vi "SubVI_TurnLeft_Auto.vi"(10 "Speed":dbl=1000.0) -> ()   [LabVIEW 2017]
uses:
  <vilib>/Rock Robotics/WPI/ThirdParty/Sensors/navX/_TypeDefs/FRIC_navX_DeviceNumbersTypeDef.ctl
  <vilib>/Rock Robotics/WPI/ThirdParty/Phoenix-LabVIEW/Motor Controller/Controls/CTRE_Phoenix_MotorControl_ControlMode.ctl
panel:
  out "Yaw":dbl
  in  "F 2":dbl=0.1
  in  "D 2":dbl=0.1
  in  "I 2":dbl
  in  "P 2":dbl=0.025
  in  "F":dbl=0.1
  in  "D":dbl=0.1
  in  "I":dbl
  in  "P":dbl=0.025
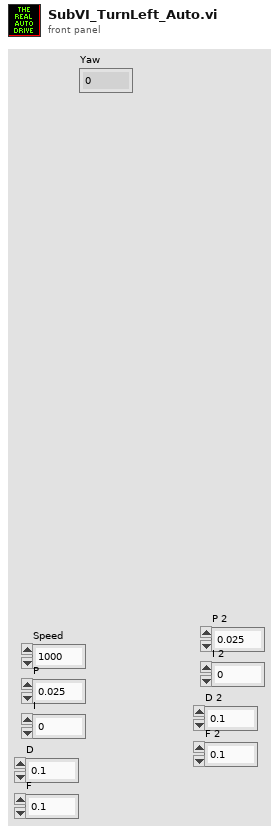
[diagram p1: front panel]
types:
  T1 = typedef "FRIC_navX_DeviceNumbersTypeDef.ctl" = enum16{"Dev0", "Dev1", "Dev2", "Dev3"}
  T2 = typedef "WPI_MotorControlDeviceRef.ctl" = cluster{"DeviceStatus":errorcluster, "Type":T3, "PWM":cluster{"PWM Channel":T4, "DeadBand":T5}, "CAN":cluster{"Device Number":u8, "SetOutput VI Ref":variant, "GetOutput VI Ref":variant, "Enable VI Ref":variant, "Disable VI Ref":variant, "Data":variant}, "Invert":bool, "DIO PWM":cluster{"PWM \"Enable\" Channel":T4, "DIOChannel":T6, "PWM Rate":dbl}}
  T3 = typedef "WPI_MotorControlType.ctl" = enum16{"PWM", "CAN", "DIO PWM"}
  T4 = typedef "FPGA_DIOPWMChannel.ctl" = enum8{"PWM 0", "PWM 1", "PWM 2", "PWM 3", "PWM 4", "PWM 5", "PWM 6", "PWM 7", "PWM 8", "PWM 9", "PWM MXP 0", "PWM MXP 1", "PWM MXP 2", "PWM MXP 3", "PWM MXP 4", "PWM MXP 5", "PWM MXP 6", "PWM MXP 7", "PWM MXP 8", "PWM MXP 9", "Invalid"}
  T5 = typedef "WPI_PWMDeadband.ctl" = cluster{"Name":string, "maxPositivePwm":i32, "minPositivePwm":i32, "centerPwm":i32, "maxNegativePwm":i32, "minNegativePwm":i32, "angularRange":u16}
  T6 = typedef "FPGA_DIOChannel.ctl" = enum8{"DIO 0", "DIO 1", "DIO 2", "DIO 3", "DIO 4", "DIO 5", "DIO 6", "DIO 7", "DIO 8", "DIO 9", "DIO MXP 0", "DIO MXP 1", "DIO MXP 2", "DIO MXP 3", "DIO MXP 4", "DIO MXP 5", "DIO MXP 6", "DIO MXP 7", "DIO MXP 8", "DIO MXP 9", "DIO MXP 10", "DIO MXP 11", "DIO MXP 12", "DIO MXP 13", "DIO MXP 14", "DIO MXP 15", "SPI Port CS1", "SPI Port CS2", "SPI Port CS3", "SPI Port MISO", "SPI Port MOSI", "Invalid"}
  T7 = cluster{"Yaw":dbl, "Roll":dbl, "Pitch":dbl, "Heading":dbl, "Fused Heading":dbl}
  T8 = typedef "CTRE_Phoenix_MotorControl_ControlMode.ctl" = u16
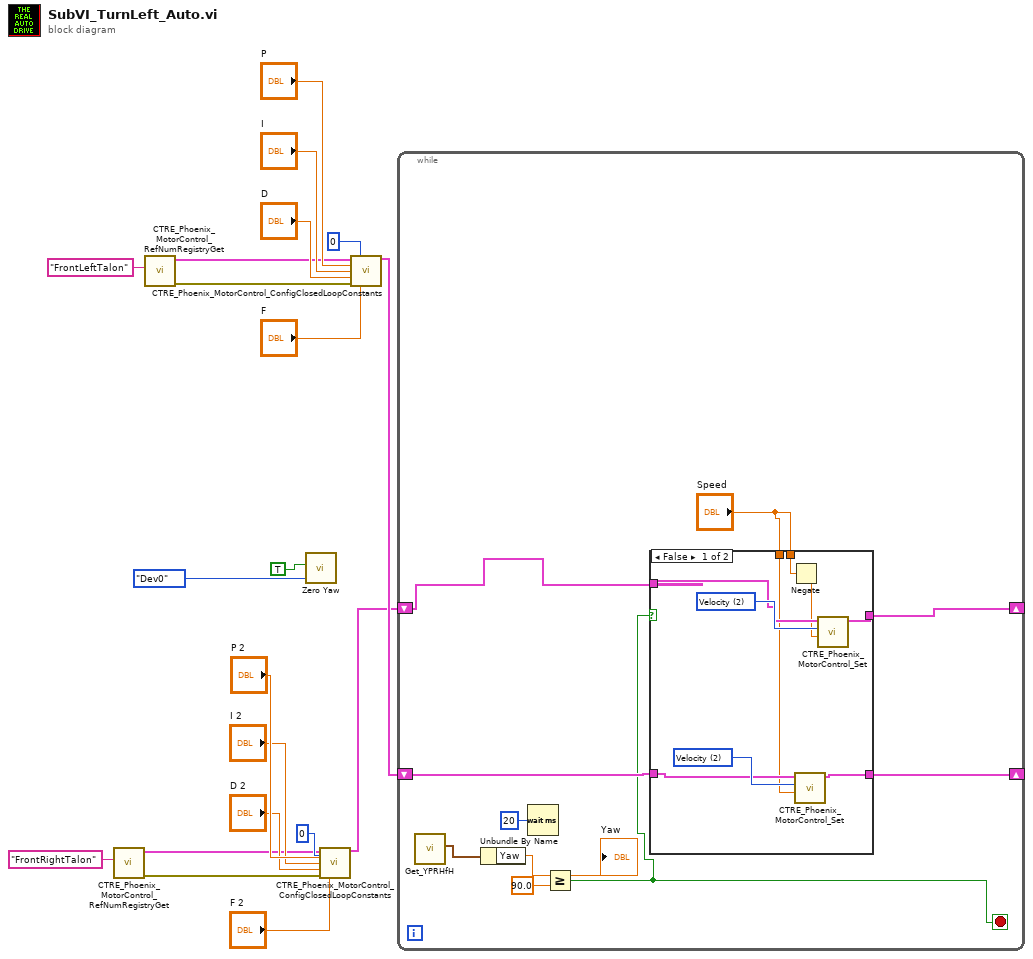
[diagram p0: block diagram]
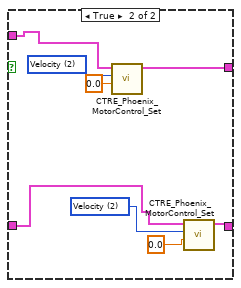
[diagram p2: hidden frame]
diagram:
  n1 = call <vilib>:"CTRE_Phoenix_MotorControl_RefNumRegistryGet.vi"("refnum name"="FrontRightTalon") -> ("error out"=w3:errorcluster, "PhoenixMotorControlDevRef"=w4:T2)  [unwired: 9 in]
  n2 = call <vilib>:"CTRE_Phoenix_MotorControl_RefNumRegistryGet.vi"("refnum name"="FrontLeftTalon") -> ("error out"=w5:errorcluster, "PhoenixMotorControlDevRef"=w6:T2)  [unwired: 9 in]
  n3 = call <vilib>:"Zero Yaw.vi"("Device Number"=FRIC_navX_DeviceNumbersTypeDef."Dev0", "Zero"=TRUE) -> ()  [unwired: 10 in]
  n4 = call <vilib>:"CTRE_Phoenix_MotorControl_ConfigClosedLoopConstants.vi"("PhoenixMotorControlDevRef"=w4, "slotIdx"=0, "P"="P 2", "I"="I 2", "D"="D 2", "error in (no error)"=w3, "F"="F 2") -> ("PhoenixMotorControlDevRef"=w7:T2)  [unwired: 7 in, 1 out]
  n5 = call <vilib>:"CTRE_Phoenix_MotorControl_ConfigClosedLoopConstants.vi"("PhoenixMotorControlDevRef"=w6, "slotIdx"=0, "P"="P", "I"="I", "D"="D", "error in (no error)"=w5, "F"="F") -> ("PhoenixMotorControlDevRef"=w16:T2)  [unwired: 7 in, 1 out]
  n6 = while {
    shift-right: [w23] -> _
    shift-left: w16 -> [w24]
    shift-right: [w30] -> _
    shift-left: w7 -> [w28]
    stop <- w22 stop-if-true
    n7 = call <vilib>:"Get_YPRHfH.vi"() -> ("YRPHfH"=w27:T7)  [unwired: 11 in]
    n8 = Unbundle By Name(w27) -> ("Yaw"=w26:dbl)
    "Yaw" <- w26
    n9 = Wait (ms)(milliseconds to wait=u32 20) -> ()  [unwired: 1 out]
    n10 = Greater Or Equal?(x=w26, y=90.0) -> (x >= y?=w22:bool)
    n11 = case shown="False" w22 {
      tunnel: [w38 w45] -> w30
      tunnel: w28 -> [w37 w44]
      tunnel: w24 -> [w35 w42]
      tunnel: [w34 w40] -> w23
      tunnel: "Speed" -> [w33 _]
      tunnel: "Speed" -> [w31 _]
      frame False {
        w36 = T8 2 items=["PercentOutput"=0, "Position"=1, "Velocity"=2, "Current"=3, "Follower"=5, "MotionProfile"=6, "MotionMagic"=7, "MotionMagicArc"=8, "MotionProfileArc"=10, "Disabled"=15] ("Control Mode")
        w39 = T8 2 items=["PercentOutput"=0, "Position"=1, "Velocity"=2, "Current"=3, "Follower"=5, "MotionProfile"=6, "MotionMagic"=7, "MotionMagicArc"=8, "MotionProfileArc"=10, "Disabled"=15] ("Control Mode")
        n12 = Negate(x=w33) -> (-x=w32:dbl)
        n13 = call <vilib>:"CTRE_Phoenix_MotorControl_Set.vi"("Output"=w31, "Control Mode"=w36, "PhoenixMotorControlDevRef"=w35) -> ("PhoenixMotorControlDevRef"=w34:T2)  [unwired: 7 in, 1 out]
        n14 = call <vilib>:"CTRE_Phoenix_MotorControl_Set.vi"("Output"=w32, "Control Mode"=w39, "PhoenixMotorControlDevRef"=w37) -> ("PhoenixMotorControlDevRef"=w38:T2)  [unwired: 7 in, 1 out]
      }
      frame True {
        w43 = T8 2 items=["PercentOutput"=0, "Position"=1, "Velocity"=2, "Current"=3, "Follower"=5, "MotionProfile"=6, "MotionMagic"=7, "MotionMagicArc"=8, "MotionProfileArc"=10, "Disabled"=15] ("Control Mode")
        w46 = T8 2 items=["PercentOutput"=0, "Position"=1, "Velocity"=2, "Current"=3, "Follower"=5, "MotionProfile"=6, "MotionMagic"=7, "MotionMagicArc"=8, "MotionProfileArc"=10, "Disabled"=15] ("Control Mode")
        n15 = call <vilib>:"CTRE_Phoenix_MotorControl_Set.vi"("Output"=0.0, "Control Mode"=w46, "PhoenixMotorControlDevRef"=w44) -> ("PhoenixMotorControlDevRef"=w45:T2)  [unwired: 7 in, 1 out]
        n16 = call <vilib>:"CTRE_Phoenix_MotorControl_Set.vi"("Output"=0.0, "Control Mode"=w43, "PhoenixMotorControlDevRef"=w42) -> ("PhoenixMotorControlDevRef"=w40:T2)  [unwired: 7 in, 1 out]
      }
    }
  }
